vi "Move piezo.vi"(4 "Canal":enum16{"X", "Y"}(ring), 6 "dV":sgl=0.4 min=0.1 max=5 step=0.1 format="%.1f", 8 "error in (no error)":errorcluster, 9 "Index":i32, 10 "Rango":u8=7 max=100 step=1, 11 "VISA Refnum in":refnum<visa-resource-name>) -> (0 "error out":errorcluster, 2 "Stop?":bool, 3 "Voltage":sgl)   [LabVIEW 2020]
doc: "Send command to piezo driver to increment its voltage. Determines if the Range voltage value has been reached; if so, sent True to Stop?."
uses:
  <vilib>/Instr/_visa.llb/VISA Configure Serial Port (Instr).vi
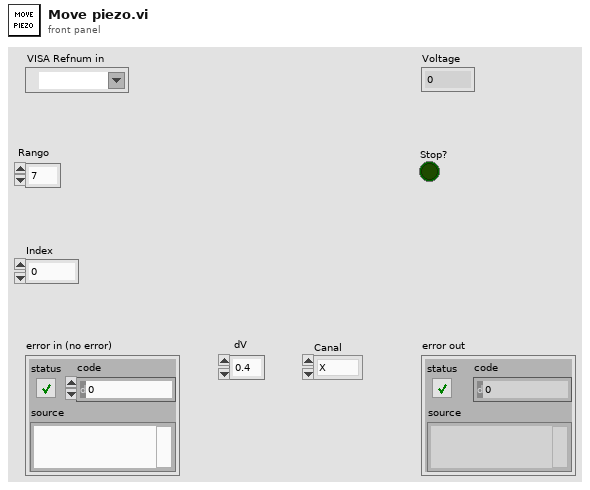
[diagram p1: front panel]
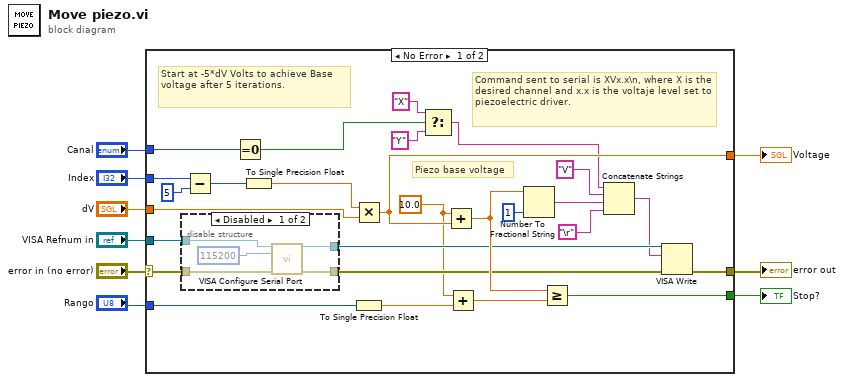
[diagram p0: block diagram]
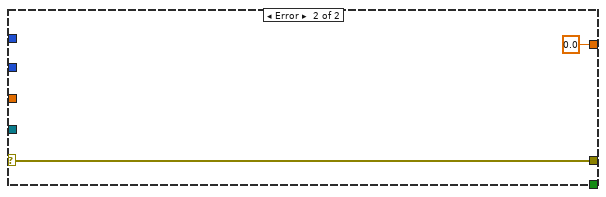
[diagram p3: hidden frame]
diagram:
  n1 = case shown="No Error" "error in (no error)" {
    selector: "error in (no error)" -> [w33 w45]
    tunnel: "Rango" -> [w36 _]
    tunnel: "dV" -> [w35 _]
    tunnel: "VISA Refnum in" -> [w34 _]
    tunnel: [w32 w45] -> w5
    tunnel: "Index" -> [w19 _]
    tunnel: [w31 _] -> w3
    tunnel: [w20 sgl 0.0] -> w2
    tunnel: "Canal" -> [w12 _]
    frame No Error {
      w15 = sgl 10.0 ("y")
      # "Start at -5*dV Volts to achieve Base voltage after 5 iterations."
      # "Piezo base voltage"
      # "Command sent to serial is XVx.x\\n, where X is the desired channel and x.x is the voltaje level set to piezoelectric driver."
      n2 = disable-structure shown="Disabled" {
        disable-tunnel: w34 -> [w41 w42]
        disable-tunnel: w33 -> [w39 w43]
        disable-tunnel: [w38 w43] -> w23
        disable-tunnel: [w37 w42] -> w22
        frame Disabled {
          n3 = call-poly "VISA Configure Serial Port"("VISA resource name"=w41, "baud rate (9600)"=u32 115200, "error in (no error)"=w39) -> ("VISA resource name out"=w37:refnum<visa-resource-name>, "error out"=w38:errorcluster)  [unwired: 11 in]
        }
        frame Enabled {
        }
      }
      n4 = Subtract(x=w19, y=5) -> (x-y=w18:i32)
      n5 = Equal To 0?(x=w12) -> (x = 0?=w11:bool)
      n6 = To Single Precision Float(number=w18) -> (single precision float=w25:sgl)
      n7 = Multiply(x=w25, y=w35) -> (x*y=w20:sgl)
      n8 = To Single Precision Float(number=w36) -> (single precision float=w24:sgl)
      n9 = Select(t="X" ("string"), s=w11, f="Y") -> (s? t:f=w10:string)
      n10 = Add(x=w15, y=w20) -> (x+y=w26:sgl)
      n11 = Add(x=w15, y=w24) -> (x+y=w16:sgl)
      n12 = Number To Fractional String(number=w26, precision (6)=i16 1) -> (F-format string=w30:string)  [unwired: 2 in]
      n13 = Greater Or Equal?(x=w26, y=w16) -> (x >= y?=w31:bool)
      n14 = Concatenate Strings(w10, "V" ("string"), w30, "\r") -> (w21:string)
      n15 = VISA Write(VISA resource name=w22, write buffer=w21, error in (no error)=w23) -> (error out=w32:errorcluster)  [unwired: 2 out]
    }
    frame Error {
    }
  }
  "error out" <- w5
  "Stop?" <- w3
  "Voltage" <- w2
